vi "WHEN.vi"(10 "argv":string[](array[string]), 11 "args":u8) -> ()   [LabVIEW 2011]
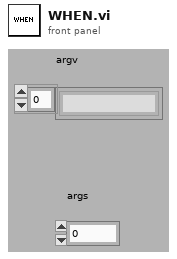
[diagram p1: front panel]
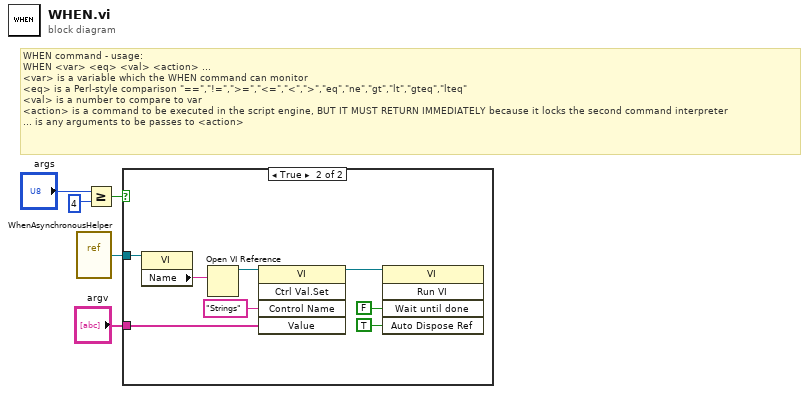
[diagram p0: block diagram]
diagram:
  # "WHEN command - usage:\nWHEN <var> <eq> <val> <action> ...\n<var> is a variable which the WHEN command can monitor\n<eq> is a Perl-style comparison \"==\",\"!=\",\">=\",\"<=\",\"<\",\">\",\"eq\",\"ne\",\"gt\",\"lt\",\"gteq\",\"lteq\"\n<val> is a number to compare to var\n<action> is a command to be executed in the script engine, BUT IT MUST RETURN IMMEDIATELY because it locks the second command interpreter\n... is any arguments to be passes to <action>"
  n1 = vi-ref "WhenAsynchronousHelper.vi"() -> (w5:refnum<vi>)
  n2 = Greater Or Equal?(x="args", y=u8 4) -> (x >= y?=w1:bool)
  n3 = case shown="True" w1 {
    tunnel: w5 -> [_ w12]
    tunnel: "argv" -> [_ w10]
    frame False {
    }
    frame True {
      n4 = property class="VI"(reference=w12) -> ("Name"=w13:string)  [unwired: 1 in, 2 out]
      n5 = Open VI Reference(vi path=w13) -> (vi reference=w11:refnum<vi>)  [unwired: 2 in, 4 out]
      n6 = invoke class="VI" method="Ctrl Val.Set"(reference=w11, "Control Name"="Strings", "Value"=w10) -> (reference out=w8:refnum<vi>)  [unwired: 2 in, 4 out]
      n7 = invoke class="VI" method="Run VI"(reference=w8, "Wait until done"=FALSE ("Wait Until Done"), "Auto Dispose Ref"=TRUE ("Auto Dispose Reference")) -> ()  [unwired: 2 in, 5 out]
    }
  }
